vi "Ping.vi"(0 "InfluxDB in":refnum<class "InfluxDB Client.lvclass">, 11 "error in (no error)":errorcluster) -> (4 "InfluxDB out":refnum<class "InfluxDB Client.lvclass">, 6 "Ping status":string, 15 "error out":errorcluster)   [LabVIEW 2013, in "InfluxDB Client.lvclass"]
doc: "Performs a ping to retrieve status information."
uses:
  InfluxDB Client.lvclass
  InfluxDB Client.lvclass/InfluxDB Client.ctl
  <vilib>/LVH/i3 JSON/JSON Parsing/Get Object Parameter Files/Get Object Parameter - String.vi
  <vilib>/httpClient/LabVIEWHTTPClient.lvlib
  <vilib>/LVH/i3 JSON/i3-json.lvlib
panel:
  out "Status":string
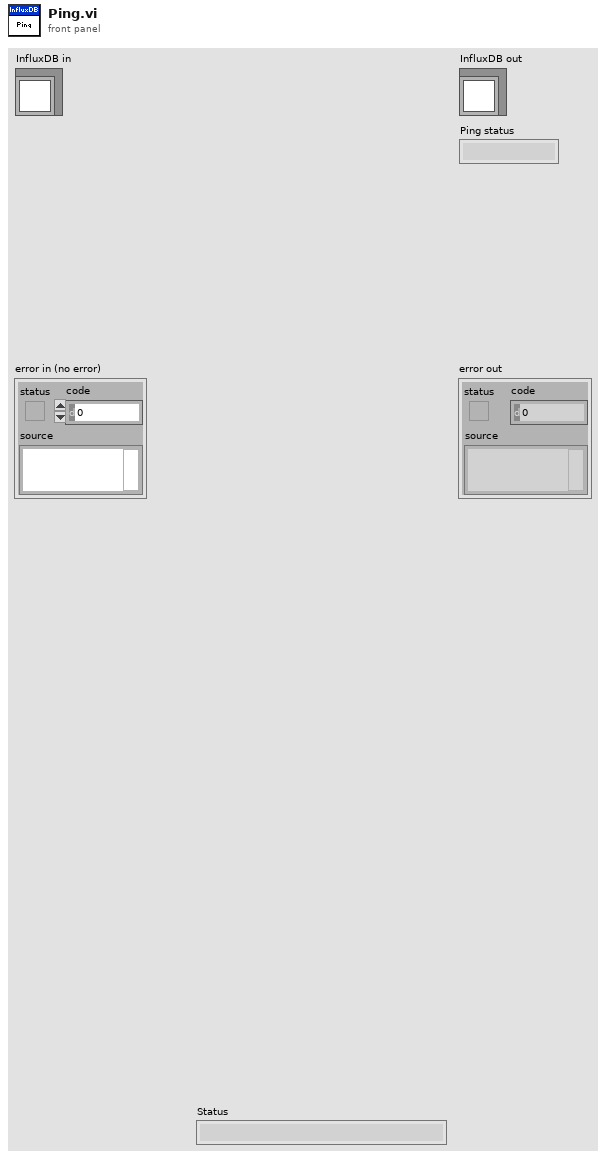
[diagram p1: front panel]
types:
  T1 = typedef "LabVIEWHTTPClient.lvlib/ClientHandle.ctl" = refnum<k1>
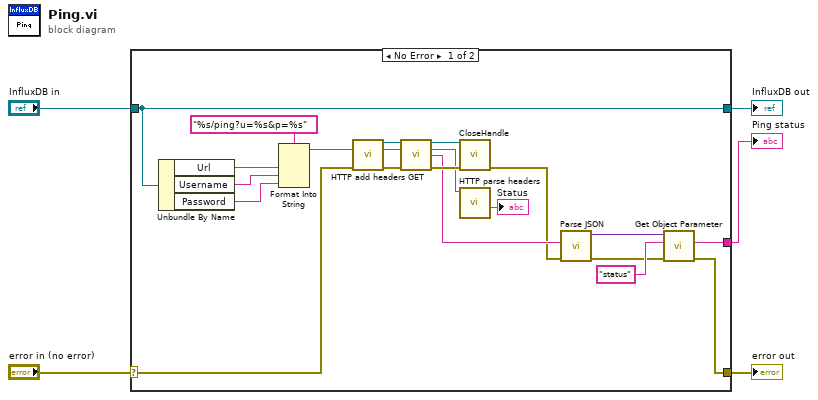
[diagram p0: block diagram]
diagram:
  n1 = case shown="No Error" "error in (no error)" {
    selector: "error in (no error)" -> [w13 w27]
    tunnel: [w7 w27] -> w4
    tunnel: [w25 w26] -> w2
    tunnel: "InfluxDB in" -> [w25 w26]
    tunnel: [w10 _] -> w1
    frame No Error {
      n2 = Unbundle By Name(w25) -> ("Url"=w23:string, "Username"=w17:string, "Password"=w16:string)
      n3 = Format Into String(format string="%s/ping?u=%s&p=%s" ("url"), w23, w17, w16) -> (resulting string=w20:string)  [unwired: 2 in, 1 out]
      n4 = call "HTTP add headers.vi"("error in (no error)"=w13) -> ("client handle out"=w15:T1, "error out"=w14:errorcluster)  [unwired: 13 in]
      n5 = call <vilib>:"GET.vi"("client handle"=w15, "url"=w20, "error in (no error)"=w14) -> ("client handle out"=w22:T1, "headers"=w19:string, "body"=w12:string, "error out"=w21:errorcluster)  [unwired: 9 in]
      n6 = call <vilib>:"CloseHandle.vi"("client handle"=w22, "error in (no error)"=w21) -> ("error out"=w6:errorcluster)  [unwired: 13 in]
      n7 = call "HTTP parse headers.vi"("HTTP headers"=w19) -> ("Status"=→"Status":string)  [unwired: 8 in, 2 out]
      n8 = call <vilib>:"Parse JSON.vi"("error in (no error)"=w6, "JSON String"=w12) -> ("error out"=w8:errorcluster, "JSON Tree"=w11:variant)  [unwired: 6 in, 2 out]
      n9 = call-poly <vilib>:"Get Object Parameter.vi"("error in (no error)"=w8, "Parameter Name"="status", "JSON Tree In (JSON Object)"=w11) -> ("error out"=w7:errorcluster, "String Value"=w10:string)  [unwired: 5 in, 2 out]
    }
    frame Error {
    }
  }
  "error out" <- w4
  "InfluxDB out" <- w2
  "Ping status" <- w1
